vi "NF LI56xx dvr sVOLTage psd1 AC RANGe AUTO ONCE.vi"(8 "error in":errorcluster caption="error in (no error)" {"code" format="%.0x"}, 11 "VISA resource name":refnum<visa-resource-name>) -> (0 "error out":errorcluster {"code" format="%.0x"}, 3 "VISA resource name copy":refnum<visa-resource-name>)   [LabVIEW 2019]
doc: "Automatically set voltage sensitivity one time. \nWhen voltage sensitivity is set automatically, dynamic reserve is also set automatically."
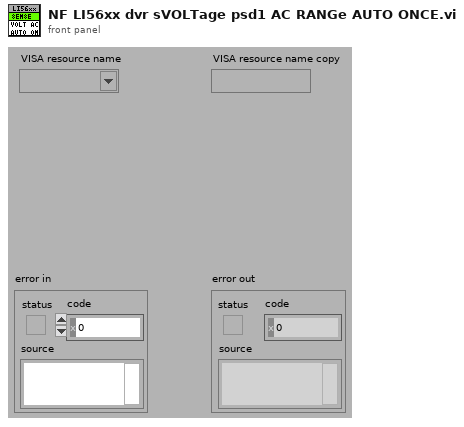
[diagram p1: front panel]
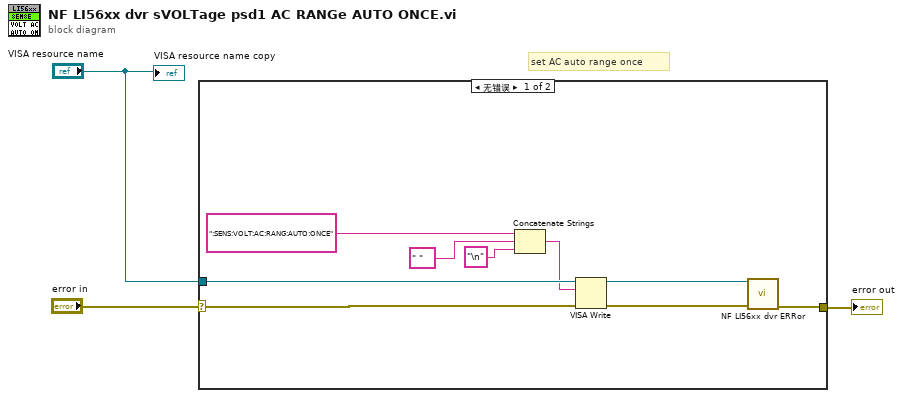
[diagram p0: block diagram]
diagram:
  # "set AC auto range once"
  n1 = case shown="无错误" "error in" {
    selector: "error in" -> [w12 w13]
    tunnel: [w8 w13] -> w3
    tunnel: "VISA resource name" -> [w11 _]
    frame No Error {
      n2 = Concatenate Strings(":SENS:VOLT:AC:RANG:AUTO:ONCE" ("•¶Žš—ñ"), " ", "\n" ("Œ`Ž®•¶Žš—ñ")) -> (w6:string)
      n3 = VISA Write(VISA resource name=w11, write buffer=w6, error in (no error)=w12) -> (VISA resource name out=w10:refnum<visa-resource-name>, error out=w9:errorcluster)  [unwired: 1 out]
      n4 = call "NF LI56xx dvr ERRor.vi"("VISA resource name"=w10, "error in (no error)"=w9) -> ("error out"=w8:errorcluster)  [unwired: 10 in, 3 out]
    }
    frame Error {
    }
  }
  "error out" <- w3
  "VISA resource name copy" <- "VISA resource name"
